vi "BRig_comm_webdav_myrioUsername.vi"() -> (2 "output_myrioUsername":string)   [LabVIEW 2014]
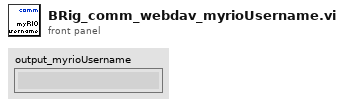
[diagram p1: front panel]
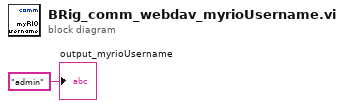
[diagram p0: block diagram]
diagram:
  "output_myrioUsername" <- "admin" ("host uri prefix")
